vi "PDashPathHistory--constant.vi"() -> (3 "PDashPathHistory":string)   [LabVIEW 2020, in "Panther Dashboard.lvlib" / "Project.lvclass"]
uses:
  Project.lvclass
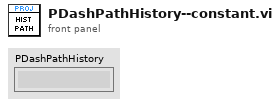
[diagram p1: front panel]
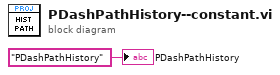
[diagram p0: block diagram]
diagram:
  "PDashPathHistory" <- "PDashPathHistory" ("key")
